vi "Skew_Image4.vi"(4 "[IN] Skewed Image":T1, 5 "[IN] Share Angle":u16 max=89 step=1, 6 "[IN] Calculation mode":enum16{"Single core", "2x cores", "4x cores"}(ring), 7 "error IN":errorcluster, 8 "[IN] Y = Array rows":i32, 9 "[IN] X = Array cols":i32, 10 "[IN] Source Image U16":u16[][](array[numeric])) -> (0 "error OUT":errorcluster, 3 "[OUT] Skewed Image":T1)   [LabVIEW 2020]
uses:
  <vilib>/vision/Image Controls.llb/IMAQ Image.ctl
  <vilib>/vision/NI_Vision_Development_Module.lvlib
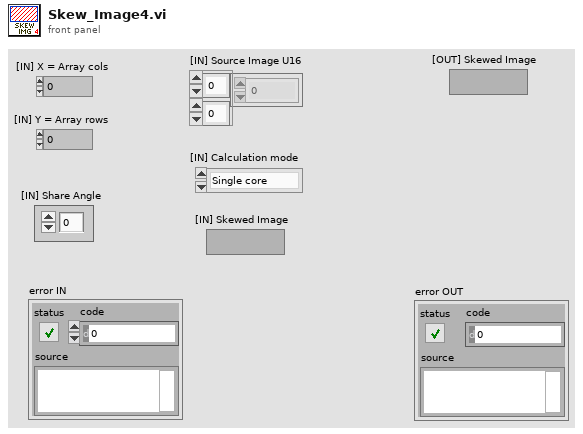
[diagram p1: front panel]
types:
  T1 = typedef "IMAQ Image.ctl" = refnum<image>
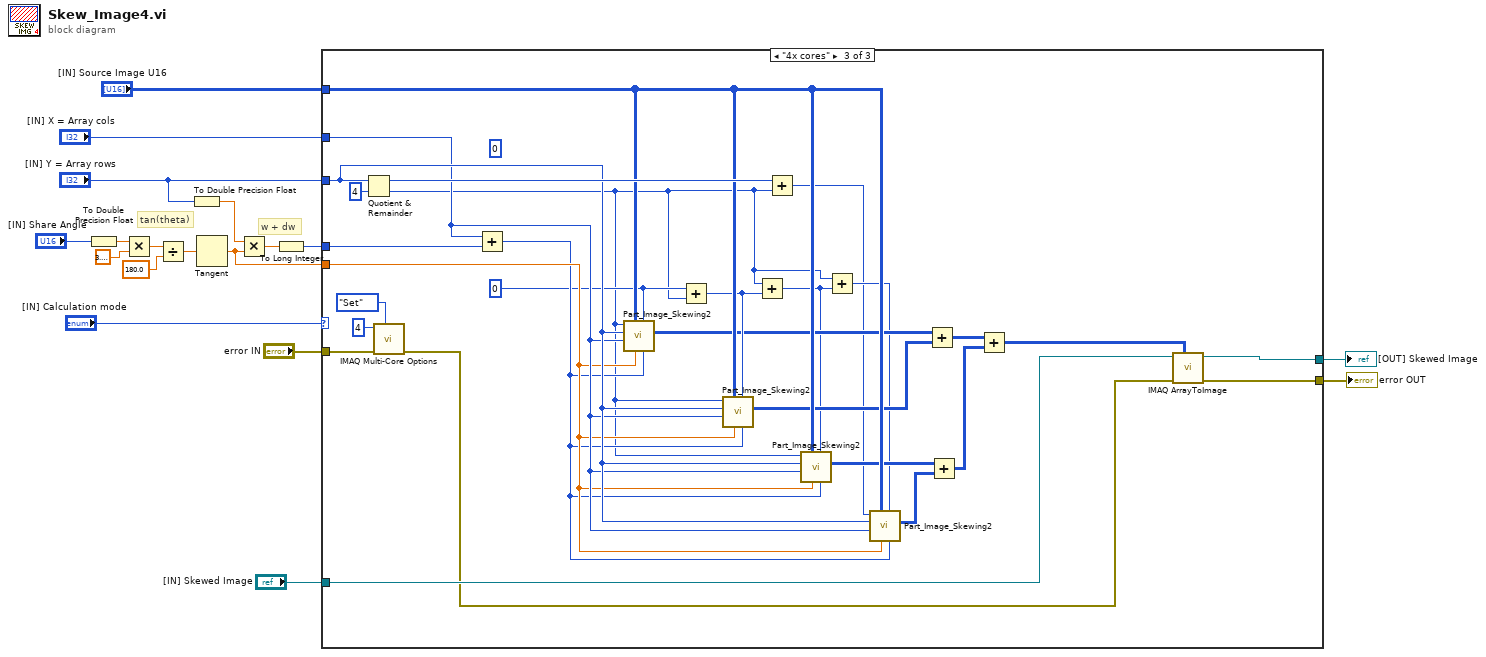
[diagram p0: block diagram]
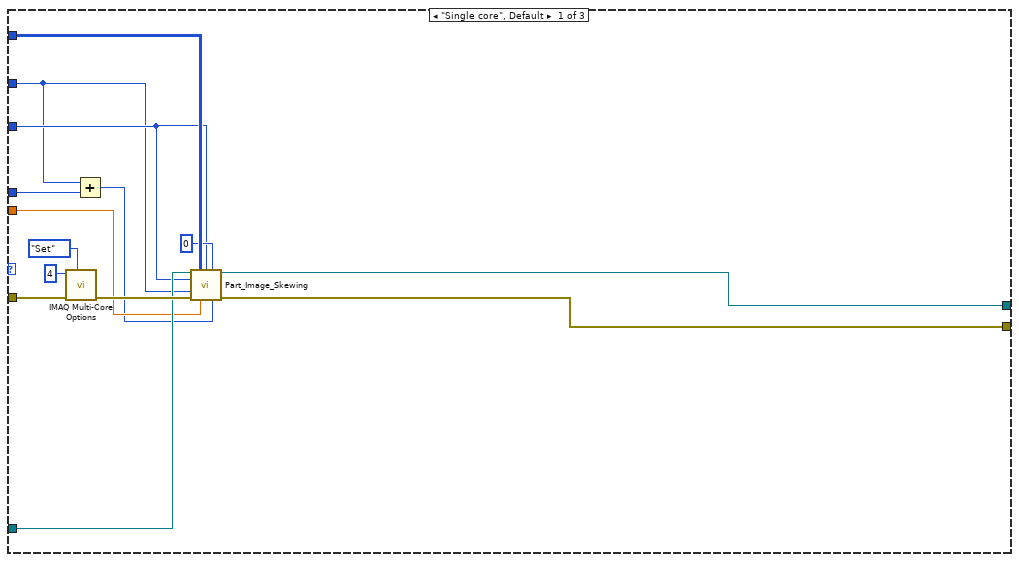
[diagram p2: hidden frame]
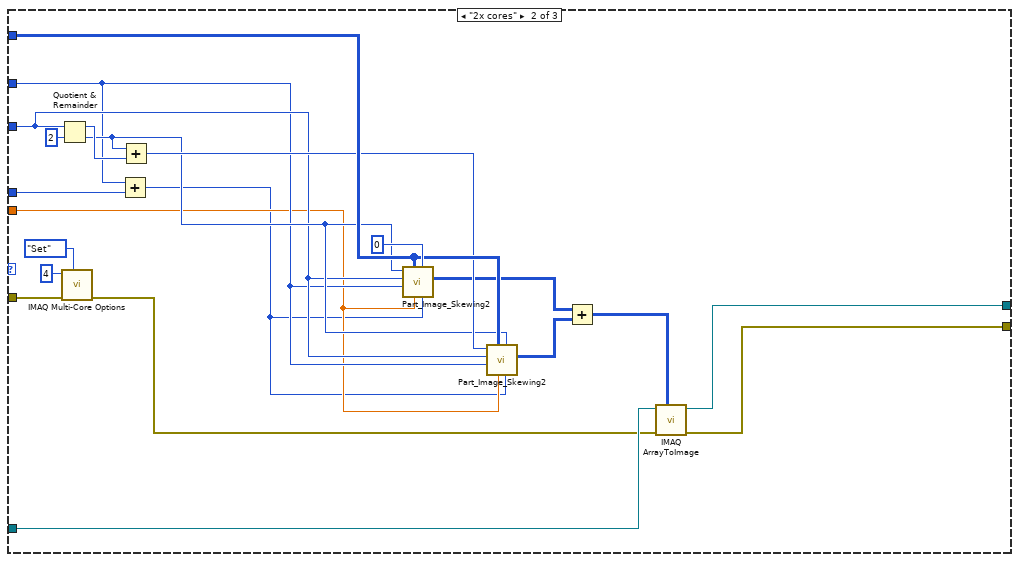
[diagram p3: hidden frame]
diagram:
  # "w + dw"
  # "tan(theta)"
  n1 = To Double Precision Float(number="[IN] Share Angle") -> (double precision float=w18:dbl)
  n2 = Multiply(x=w18, y=3.141592653589793) -> (x*y=w17:dbl)
  n3 = Divide(x=w17, y=180.0) -> (x/y=w15:dbl)
  n4 = To Double Precision Float(number="[IN] Y = Array rows") -> (double precision float=w9:dbl)
  n5 = Tangent(1:w15) -> (0:w13:dbl)
  n6 = Multiply(x=w9, y=w13) -> (x*y=w12:dbl)
  n7 = To Long Integer(number=w12) -> (32bit integer=w14:i32)
  n8 = case shown="\"4x cores\"" "[IN] Calculation mode" {
    tunnel: w14 -> [w22 w52 w80]
    tunnel: w13 -> [w20 w41 w72]
    tunnel: "[IN] Source Image U16" -> [w27 w46 w75]
    tunnel: "[IN] X = Array cols" -> [w21 w42 w73]
    tunnel: "[IN] Y = Array rows" -> [w23 w43 w74]
    tunnel: "error IN" -> [w30 w48 w77]
    tunnel: [w24 w33 w69] -> w3
    tunnel: [w25 w34 w70] -> w2
    tunnel: "[IN] Skewed Image" -> [w28 w37 w68]
    frame "Single core", Default {
      n9 = call "IMAQ Multi-Core Options"("Get/Set Number of Cores (Get)"=enum32{"Get", "Set", "Set Max Available"}."Set", "error in (no error)"=w30, "Specified Number of Cores"=u32 4) -> ("error out"=w29:errorcluster)  [unwired: 7 in, 1 out]
      n10 = Add(x=w21, y=w22) -> (x+y=w19:i32)
      n11 = call "Part_Image_Skewing.vi"("[IN] Part Image"=w28, "[IN] Source Image U16"=w27, "[IN] Rows Part"=w23, "[IN] Part shift"=0, "[IN] Rows"=w23, "[IN] Cols Initial"=w21, "error IN"=w29, "[IN] tan(theta)"=w20, "[IN] Cols"=w19) -> ("[OUT] Part Image"=w25:T1, "error OUT"=w24:errorcluster)  [unwired: 5 in]
    }
    frame "2x cores" {
      n12 = Quotient & Remainder(x=w43, y=2) -> (x-y*floor(x/y)=w51:i32, floor(x/y)=w44:i32)
      n13 = call "IMAQ Multi-Core Options"("Get/Set Number of Cores (Get)"=enum32{"Get", "Set", "Set Max Available"}."Set", "error in (no error)"=w48, "Specified Number of Cores"=u32 4) -> ("error out"=w36:errorcluster)  [unwired: 7 in, 1 out]
      n14 = Add(x=w42, y=w52) -> (x+y=w40:i32)
      n15 = Add(x=w44, y=w51) -> (x+y=w45:i32)
      n16 = call "Part_Image_Skewing2.vi"("[IN] Cols"=w40, "[IN] Part shift"=0, "[IN] tan(theta)"=w41, "[IN] Source Image U16"=w46, "[IN] Cols Initial"=w42, "[IN] Rows"=w43, "[IN] Rows Part"=w44) -> ("[OUT] Pixel part"=w39:u16[][])  [unwired: 4 in]
      n17 = call "Part_Image_Skewing2.vi"("[IN] Cols"=w40, "[IN] Part shift"=w44, "[IN] tan(theta)"=w41, "[IN] Source Image U16"=w46, "[IN] Cols Initial"=w42, "[IN] Rows"=w43, "[IN] Rows Part"=w45) -> ("[OUT] Pixel part"=w38:u16[][])  [unwired: 4 in]
      n18 = Add(x=w39, y=w38) -> (x+y=w35:u16[][])
      n19 = call "IMAQ ArrayToImage"("Image Pixels (U16)"=w35, "error in (no error)"=w36, "Image"=w37) -> ("error out"=w33:errorcluster, "Image Out"=w34:T1)  [unwired: 7 in]
    }
    frame "4x cores" {
      w66 = 0 ("[IN] Part shift")
      (unwired) u16 0
      n20 = Quotient & Remainder(x=w74, y=4) -> (x-y*floor(x/y)=w76:i32, floor(x/y)=w56:i32)
      n21 = call "IMAQ Multi-Core Options"("Get/Set Number of Cores (Get)"=enum32{"Get", "Set", "Set Max Available"}."Set", "error in (no error)"=w77, "Specified Number of Cores"=u32 4) -> ("error out"=w67:errorcluster)  [unwired: 7 in, 1 out]
      n22 = Add(x=w73, y=w80) -> (x+y=w71:i32)
      n23 = call "Part_Image_Skewing2.vi"("[IN] Cols"=w71, "[IN] Part shift"=w66, "[IN] tan(theta)"=w72, "[IN] Source Image U16"=w75, "[IN] Cols Initial"=w73, "[IN] Rows"=w74, "[IN] Rows Part"=w56) -> ("[OUT] Pixel part"=w64:u16[][])  [unwired: 4 in]
      n24 = Add(x=w66, y=w56) -> (x+y=w65:i32)
      n25 = call "Part_Image_Skewing2.vi"("[IN] Cols"=w71, "[IN] Part shift"=w65, "[IN] tan(theta)"=w72, "[IN] Source Image U16"=w75, "[IN] Cols Initial"=w73, "[IN] Rows"=w74, "[IN] Rows Part"=w56) -> ("[OUT] Pixel part"=w63:u16[][])  [unwired: 4 in]
      n26 = Add(x=w56, y=w65) -> (x+y=w57:i32)
      n27 = Add(x=w76, y=w56) -> (x+y=w54:i32)
      n28 = call "Part_Image_Skewing2.vi"("[IN] Cols"=w71, "[IN] Part shift"=w57, "[IN] tan(theta)"=w72, "[IN] Source Image U16"=w75, "[IN] Cols Initial"=w73, "[IN] Rows"=w74, "[IN] Rows Part"=w56) -> ("[OUT] Pixel part"=w62:u16[][])  [unwired: 4 in]
      n29 = Add(x=w56, y=w57) -> (x+y=w55:i32)
      n30 = call "Part_Image_Skewing2.vi"("[IN] Cols"=w71, "[IN] Part shift"=w55, "[IN] tan(theta)"=w72, "[IN] Source Image U16"=w75, "[IN] Cols Initial"=w73, "[IN] Rows"=w74, "[IN] Rows Part"=w54) -> ("[OUT] Pixel part"=w61:u16[][])  [unwired: 4 in]
      n31 = Add(x=w64, y=w63) -> (x+y=w60:u16[][])
      n32 = Add(x=w62, y=w61) -> (x+y=w59:u16[][])
      n33 = Add(x=w60, y=w59) -> (x+y=w58:u16[][])
      n34 = call "IMAQ ArrayToImage"("Image Pixels (U16)"=w58, "error in (no error)"=w67, "Image"=w68) -> ("error out"=w69:errorcluster, "Image Out"=w70:T1)  [unwired: 7 in]
    }
  }
  "error OUT" <- w3
  "[OUT] Skewed Image" <- w2
